vi "Get configuration chain.vi"(8 "error in (no error)":errorcluster, 11 "DAQMH121119OrcaFlashBase in":refnum<class "DAQOrcaFlash.lvclass">) -> (0 "error out":errorcluster, 1 "class name":string[](array[string]), 2 "configuration chain":variant[](array[variant]), 3 "DAQMH121119OrcaFlashBase out":refnum<class "DAQOrcaFlash.lvclass">)   [LabVIEW 2012, in "DAQOrcaFlash.lvclass"]
doc: "Returns an array of variants containing the configuration clusters of each class in the inheritance chain (lowest child class first), together with an array of all class names in the inheritance chain.\n\nFor classes without configuration cluster, the configuration chain contains empty variants."
uses:
  DAQOrcaFlash.lvclass
  <vilib>/Distrio/Murmex/Murmex/Murmex.lvclass
  DAQOrcaFlash.lvclass/DAQOrcaFlash.ctl
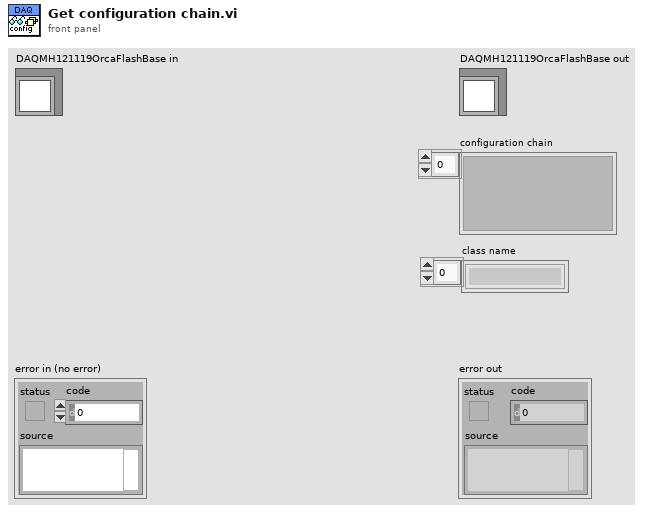
[diagram p1: front panel]
types:
  T1 = typedef "DAQOrcaFlash.lvclass/configuration_cluster.ctl" = cluster{"filepath":path, "Trigger source":T2, "Trigger mode":T3, "Sensor mode":T4, "Read out direction":T5, "Output trigger type":T6, "Output trigger source":T7, "Output trigger period":sgl[unit], "start_stop_targets":string[], "Output trigger connector":T8, "Stack component":string, "Tomo component":string, "auxiliary folder path":path, "wait before acquisition":dbl[unit], "maximum window size":i32, "final conversion folder":path}
  T2 = typedef "DAQOrcaFlash.lvclass/trigger_source.ctl" = sgl
  T3 = typedef "DAQOrcaFlash.lvclass/trigger_mode.ctl" = sgl
  T4 = typedef "DAQOrcaFlash.lvclass/sensor_mode.ctl" = sgl
  T5 = typedef "DAQOrcaFlash.lvclass/read out direction.ctl" = sgl
  T6 = typedef "DAQOrcaFlash.lvclass/output trigger type.ctl" = sgl
  T7 = typedef "DAQOrcaFlash.lvclass/output trigger source.ctl" = sgl
  T8 = typedef "DAQOrcaFlash.lvclass/connector.ctl" = enum32{"1", "2", "3"}
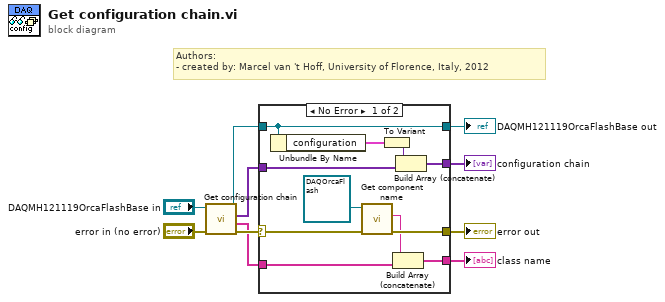
[diagram p0: block diagram]
diagram:
  # "Authors: \n- created by: Marcel van 't Hoff, University of Florence, Italy, 2012"
  n1 = call-parent "Get configuration chain.vi"("error in (no error)"="error in (no error)", "MurmexBase in"="DAQMH121119OrcaFlashBase in") -> ("error out"=w8:errorcluster, "class name"=w5:string[], "configuration chain"=w6:variant[], "MurmexBase out"=w7:refnum<class "DAQOrcaFlash.lvclass">)  [unwired: 6 in]
  n2 = case shown="No Error" w8 {
    selector: w8 -> [w21 w25]
    tunnel: [w20 w25] -> w3
    tunnel: [w12 w24] -> w2
    tunnel: w7 -> [w12 w24]
    tunnel: [w18 w23] -> w4
    tunnel: [w17 w22] -> w1
    tunnel: w6 -> [w16 w22]
    tunnel: w5 -> [w15 w23]
    frame No Error {
      n3 = Unbundle By Name(w12) -> ("configuration"=w14:T1)
      n4 = call <vilib>:"Get component name.vi"("error in (no error)"=w21, "Murmex in"=refnum<class "DAQOrcaFlash.lvclass"> refnum ("DAQMH121119OrcaFlash.lvclass")) -> ("error out"=w20:errorcluster, "component name"=w19:string)  [unwired: 7 in, 1 out]
      n5 = To Variant(anything=w14) -> (Variant=w13:variant)
      n6 = Build Array (concatenate)(w19, w15) -> (w18:string[])
      n7 = Build Array (concatenate)(w13, w16) -> (w17:variant[])
    }
    frame Error {
    }
  }
  "error out" <- w3
  "DAQMH121119OrcaFlashBase out" <- w2
  "configuration chain" <- w1
  "class name" <- w4
